vi "Set w4lvgrpc_Msg_ToServer_4.vi"(7 "Complete Call (T)":bool=TRUE, 8 "error in (no error)":errorcluster, 10 "package_templatemessage":T1, 11 "gRPCid":T2) -> (0 "error out":errorcluster)   [LabVIEW 2019, in "Generated_server.lvlib"]
uses:
  Generated_server.lvlib
  <vilib>/gRPC/LabVIEW gRPC Library/grpc-lvsupport-release.lvlib
  dcc74a39-081a-4bdd-860b-8ed792803c96.vi
  w4lvgrpc_Msg_ToServer_4_Flat.ctl
  <vilib>/gRPC/LabVIEW gRPC Library/Shared/grpcId.ctl
  w4lvgrpc_Msg_ToServer_4.ctl
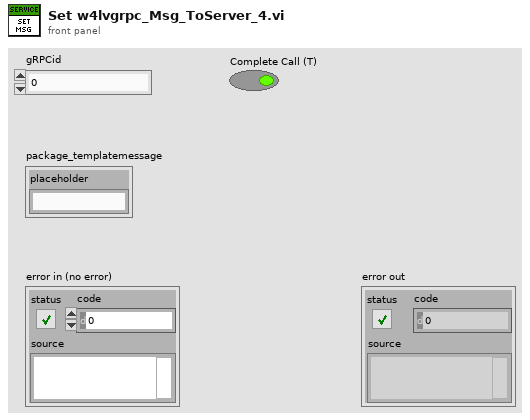
[diagram p1: front panel]
types:
  T1 = typedef "Generated_server.lvlib/w4lvgrpc_Msg_ToServer_4.ctl" = cluster{"placeholder":string}
  T2 = typedef "grpc-lvsupport-release.lvlib/grpcId.ctl" = u64
  T3 = typedef "Generated_server.lvlib/w4lvgrpc_Msg_ToServer_4_Flat.ctl" = cluster{"placeholder":string}
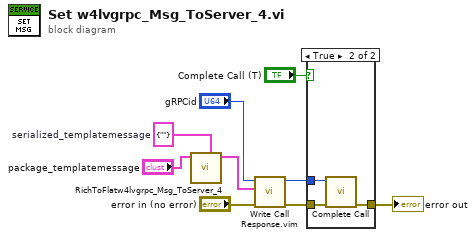
[diagram p0: block diagram]
diagram:
  w2 = T3 {"placeholder"=""}  # serialized_templatemessage
  n1 = call "RichToFlatw4lvgrpc_Msg_ToServer_4.vi"("OutputClusterType"=w2, "InputCluster"="package_templatemessage") -> ("OutputCluster"=w1:T3)  [unwired: 9 in]
  n2 = call "Write Call Response.vim"("error in"="error in (no error)", "Response Data"=w1, "gRPCid in"="gRPCid") -> ("error out"=w6:errorcluster, "gRPCid out"=w7:T2)  [unwired: 7 in]
  n3 = case shown="True" "Complete Call (T)" {
    tunnel: [w10 w13] -> w9
    tunnel: w7 -> [_ w12]
    tunnel: w6 -> [w10 w11]
    frame False {
    }
    frame True {
      n4 = call <vilib>:"Complete Call.vi"("gRPCid"=w12, "error in"=w11) -> ("error out"=w13:errorcluster)  [unwired: 8 in]
    }
  }
  "error out" <- w9
